vi "Project Name to GID.vi"(10 "Projects in":T1(array[cluster]), 11 "Name":string) -> (3 "gid":string)   [LabVIEW 2016, in "Asana.lvclass"]
uses:
  Asana.lvclass
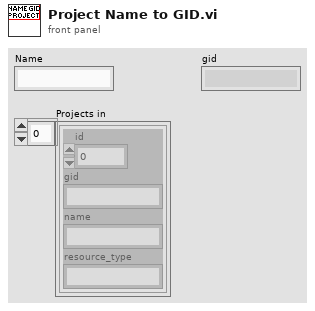
[diagram p1: front panel]
types:
  T1 = cluster{"id":i32, "gid":string, "name":string, "resource_type":string}[]
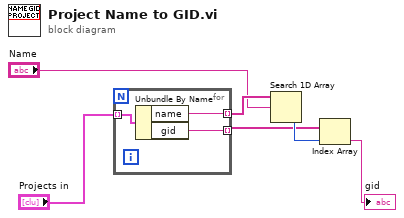
[diagram p0: block diagram]
diagram:
  n1 = for {
    tunnel: "Projects in" -> [w9] mode=indexing
    tunnel: [w8] -> w5 mode=indexing
    tunnel: [w7] -> w1 mode=indexing
    n2 = Unbundle By Name(w9) -> ("name"=w8:string, "gid"=w7:string)
  }
  n3 = Search 1D Array(1D array=w5, element="Name") -> (index of element=w2:i32)  [unwired: 1 in]
  n4 = Index Array(array=w1, index=w2) -> (element=→"gid":string)
